vi "04.1 Property Node with Event-driven SM.vi"() -> ()   [LabVIEW 2019]
uses:
  Support Files/02.4 DAQmx Configuration Cluster.ctl
  Support Files/03.2 States.ctl
  Support Files/03.2 State Machine Data.ctl
  <vilib>/DAQmx/write.llb/DAQmx Write (Analog DBL 1Chan 1Samp).vi
  <vilib>/Utility/file.llb/Write Delimited Spreadsheet (string).vi
  <vilib>/Utility/file.llb/Write Delimited Spreadsheet (DBL).vi
  <vilib>/DAQmx/create/channels.llb/DAQmx Create Channel (AO-Voltage-Basic).vi
  <vilib>/DAQmx/miscellaneous.llb/DAQmx Fill In Error Info.vi
panel:
  in  "DAQmx Configuration Cluster":T1={"Desired Sample Rate (Hz)"=-1.0, "sample mode"=10178, "Minimum value"=-1.0, "Maximum value"=-1.0, "Physical Channel"="", "units"=10143, "thermocouple type"=10072, "Samples per Channel"=0} {"thermocouple type" items=["J"=10072, "K"=10073, "N"=10077, "R"=10082, "S"=10085, "T"=10086, "B"=10047, "E"=10055]; "units" items=["Deg C"=10143, "Deg F"=10144, "Kelvins"=10325, "Deg R"=10145, "From Custom Scale"=10065]; "sample mode" items=["Finite Samples"=10178, "Continuous Samples"=10123, "Hardware Timed Single Point"=12522]}
  in  "Threshold (RMS)":dbl
  in  "Generate Stimulus":bool
  in  "Stop":bool
  in  "Clear":bool
  in  "Acquire":bool
  out "Graph":dbl[][](graph)
  out "Thershold Exceeded?":bool
  out "RMS Result per Channel":dbl[](array[numeric])
  # "ANALYSIS"
  # "EVENTS"
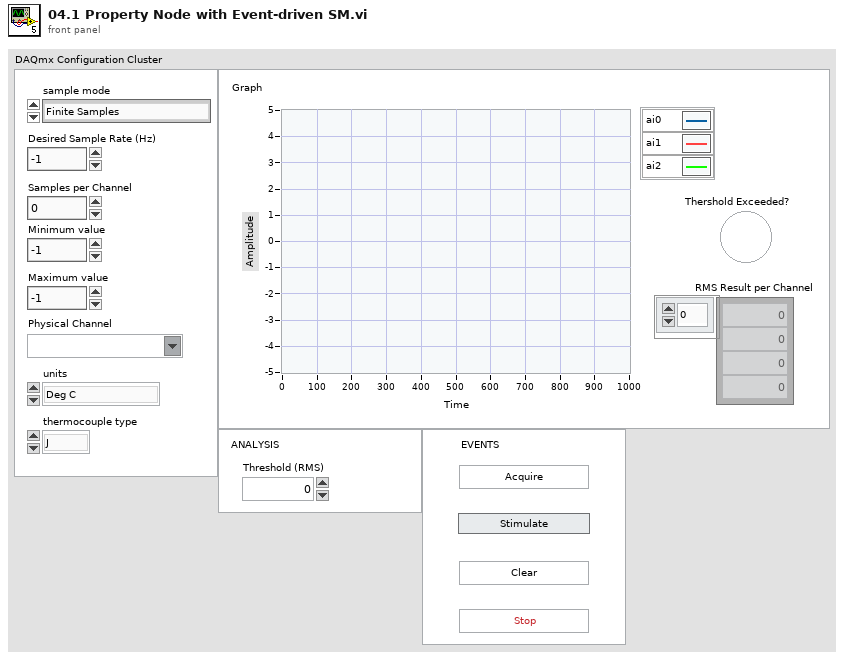
[diagram p1: front panel]
types:
  T1 = typedef "02.4 DAQmx Configuration Cluster.ctl" = cluster{"Desired Sample Rate (Hz)":dbl, "sample mode":i32, "Minimum value":dbl, "Maximum value":dbl, "Physical Channel":tag, "units":i32, "thermocouple type":i32, "Samples per Channel":i32}
  T2 = typedef "03.2 State Machine Data.ctl" = cluster{"Acquisition Data":dbl[][], "Stimulus?":bool}
  T3 = typedef "03.2 States.ctl" = enum16{"Initialize", "Update UI", "Update Stimulus", "Wait for event", "Acquire", "Analyze", "Log", "Clear", "Shutdown"}
  T4 = enum8{"Enabled", "Disabled", "Disabled and Grayed Out"}
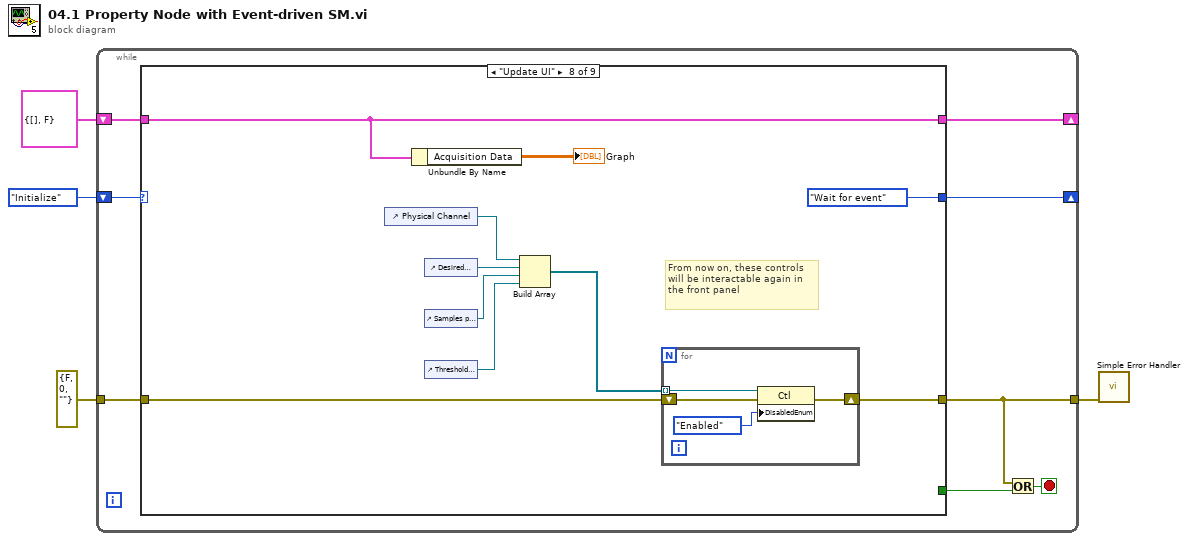
[diagram p0: block diagram]
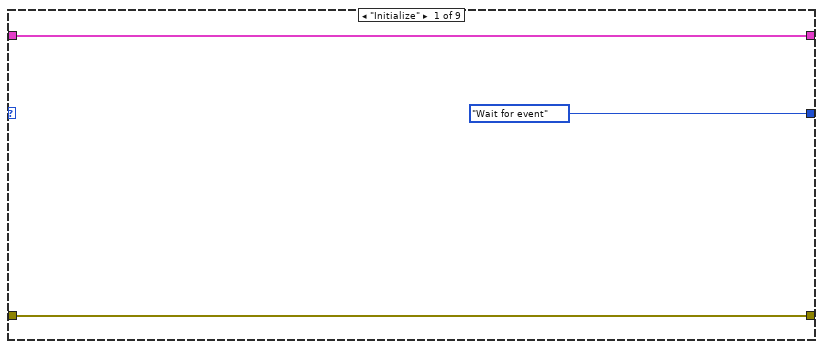
[diagram p2: hidden frame]
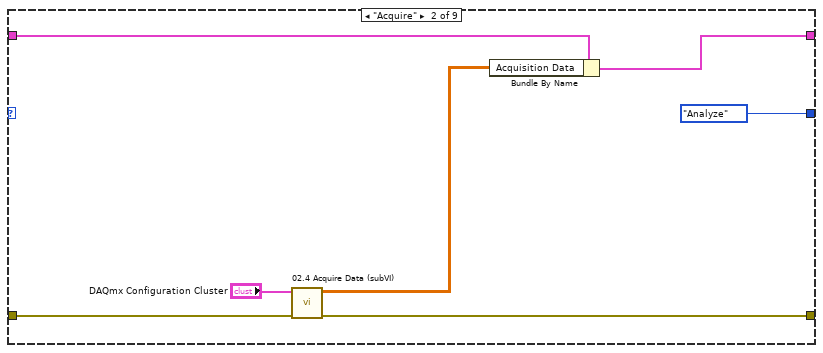
[diagram p3: hidden frame]
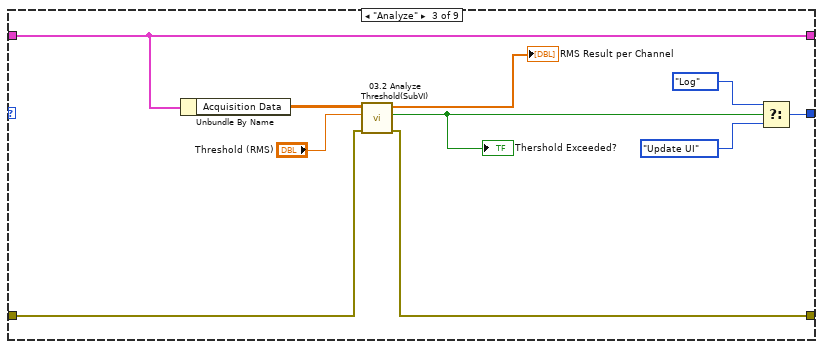
[diagram p4: hidden frame]
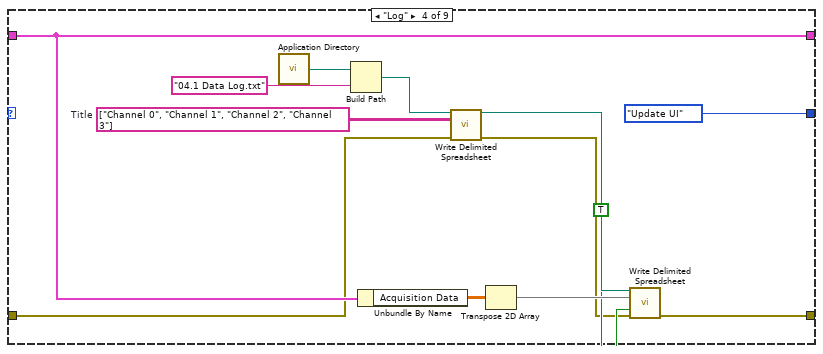
[diagram p5: hidden frame]
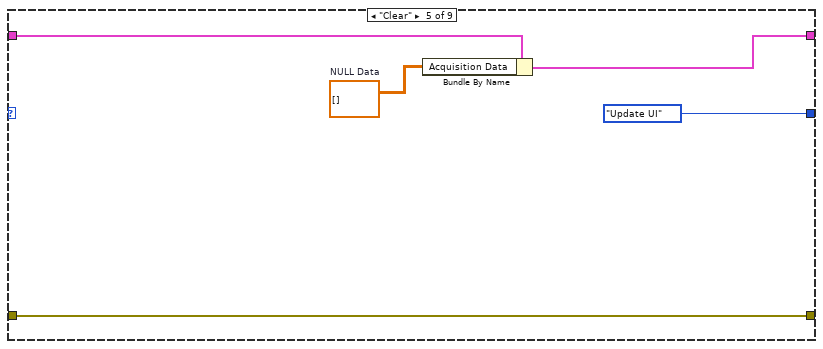
[diagram p6: hidden frame]
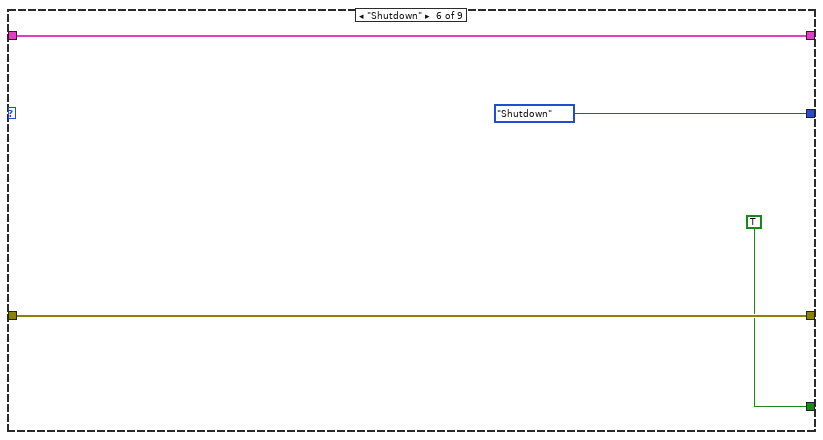
[diagram p7: hidden frame]
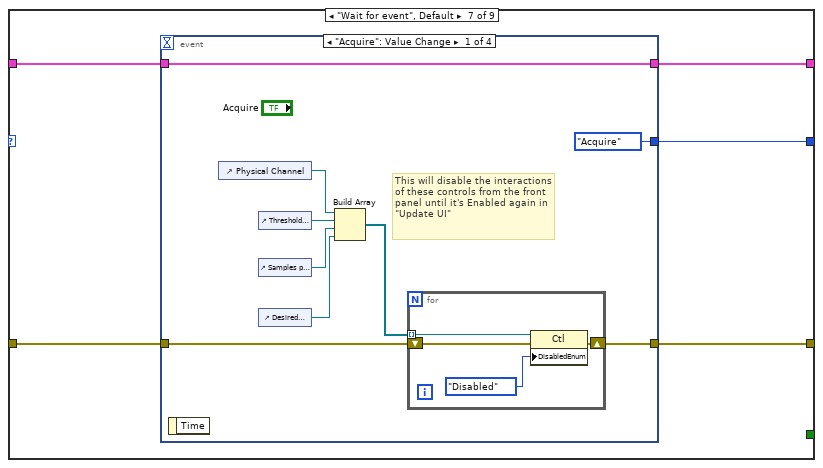
[diagram p8: hidden frame]
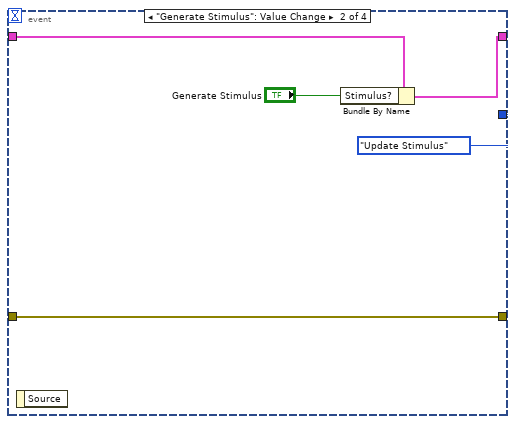
[diagram p9: hidden frame]
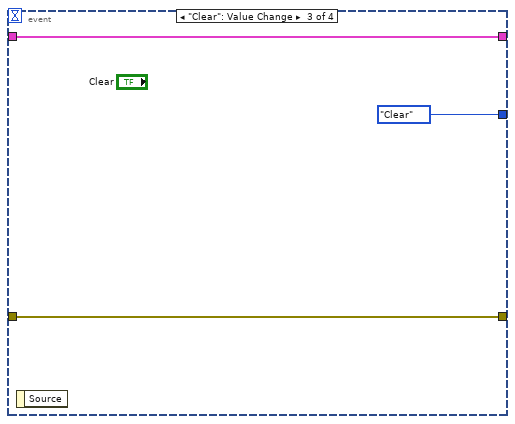
[diagram p10: hidden frame]
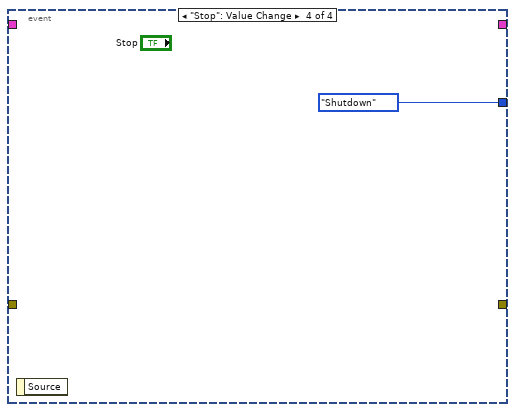
[diagram p11: hidden frame]
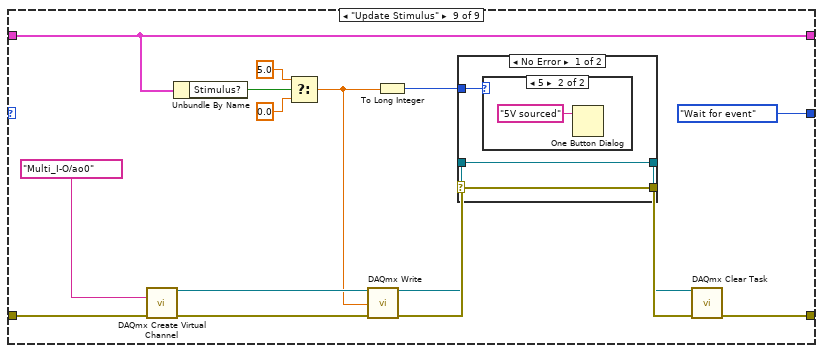
[diagram p12: hidden frame]
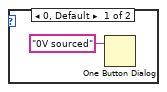
[diagram p13: hidden frame]
diagram:
  n1 = while {
    shift-right: [w11] -> _
    shift-left: 03.2_States."Initialize" ("State") -> [w12]
    tunnel: errorcluster {"status"=FALSE, "code"=0, "source"=""} ("error constant") -> [w10]
    tunnel: [w8] -> w2
    shift-right: [w7] -> _
    shift-left: T2 {"Acquisition Data"=[], "Stimulus?"=FALSE} -> [w6]
    stop <- w9 stop-if-true
    n2 = case shown="\"Update UI\"" w12 {
      tunnel: [03.2_States."Wait for event" ("State") 03.2_States."Analyze" ("State") w31 03.2_States."Update UI" ("State") 03.2_States."Update UI" ("State") 03.2_States."Shutdown" ("State") w59 03.2_States."Wait for event" ("State") 03.2_States."Wait for event" ("State")] -> w11
      tunnel: [w14 w18 w26 w43 w46 w52 w58 w87 w100] -> w8
      tunnel: w10 -> [w14 w19 w27 w33 w46 w52 w57 w86 w111]
      tunnel: [w15 w21 w25 w41 w49 w53 w56 w91 w97] -> w7
      tunnel: w6 -> [w15 w22 w25 w41 w50 w53 w55 w91 w97]
      tunnel: [_ _ _ _ _ TRUE _ _ _] -> w5
      frame "Initialize" {
      }
      frame "Acquire" {
        n3 = call "02.4 Acquire Data (subVI).vi"("Error In"=w19, "DAQmx Configuration Cluster"="DAQmx Configuration Cluster") -> ("error out"=w18:errorcluster, "2D DBL"=w20:dbl[][])  [unwired: 8 in]
        n4 = Bundle By Name(cluster=w22, "Acquisition Data"=w20) -> (w21:T2)
      }
      frame "Analyze" {
        n5 = Unbundle By Name(w25) -> ("Acquisition Data"=w32:dbl[][])
        n6 = call "03.2 Analyze Threshold(SubVI).vi"("Error In"=w27, "Threshold (RMS)"="Threshold (RMS)", "Data"=w32) -> ("Error Out"=w26:errorcluster, "Threshold exceeded?"=w28:bool, "RMS Results per Channel"=→"RMS Result per Channel":dbl[])  [unwired: 6 in]
        "Thershold Exceeded?" <- w28
        n7 = Select(t=03.2_States."Log" ("State"), s=w28, f=03.2_States."Update UI" ("State")) -> (s? t:f=w31:T3)
      }
      frame "Log" {
        w35 = string[][] [["Channel 0", "Channel 1", "Channel 2", "Channel 3"]]  # Title
        n8 = call <vilib>:"Application Directory.vi"() -> ("Application Directory"=w45:path)
        n9 = Build Path(base path=w45, name or relative path="04.1 Data Log.txt") -> (appended path=w36:path)
        n10 = Unbundle By Name(w41) -> ("Acquisition Data"=w40:dbl[][])
        n11 = call-poly <vilib>:"Write Delimited Spreadsheet.vi"("file path (dialog if empty)"=w36, "2D data"=w35, "error in (no error)"=w33) -> ("new file path (Not A Path if cancelled)"=w38:path, "error out"=w34:errorcluster)  [unwired: 11 in]
        n12 = Transpose 2D Array(2D array=w40) -> (transposed array=w39:dbl[][])
        n13 = call-poly <vilib>:"Write Delimited Spreadsheet.vi"("file path (dialog if empty)"=w38, "2D data"=w39, "append to file? (new file:F)"=TRUE, "error in (no error)"=w34) -> ("error out"=w43:errorcluster)  [unwired: 10 in, 1 out]
      }
      frame "Clear" {
        w48 = dbl[][] []  # NULL Data
        n14 = Bundle By Name(cluster=w50, "Acquisition Data"=w48) -> (w49:T2)
      }
      frame "Shutdown" {
      }
      frame "Wait for event", Default {
        n15 = event shown="[0] \"Acquire\": Value Change" {
          selector: _ -> [_ _ _ _]
          dyn-events: _ -> [_ _ _ _]
          timeout: _ -> [_ _ _ _]
          tunnel: [03.2_States."Acquire" ("State") 03.2_States."Update Stimulus" ("State") 03.2_States."Clear" ("State") 03.2_States."Shutdown" ("State")] -> w59
          tunnel: [w60 w73 w78 _] -> w58
          tunnel: w57 -> [w61 w73 w78 _]
          tunnel: [w67 w75 w80 _] -> w56
          tunnel: w55 -> [w67 w77 w80 _]
          event "Acquire": Value Change {
            # "This will disable the interactions of these controls from the front panel until it's Enabled again in \"Update UI\""
            n16 = event-data() -> ()  [unwired: 1 in, 1 out]
            n17 = control-ref of="Physical Channel"() -> (w66:refnum<vi>)
            n18 = control-ref of="Threshold (RMS)"() -> (w65:refnum<vi>)
            n19 = control-ref of="Samples per Channel"() -> (w64:refnum<vi>)
            n20 = control-ref of="Desired Sample Rate (Hz)"() -> (w63:refnum<vi>)
            n21 = Build Array(w66, w65, w64, w63) -> (w62:refnum<vi>[])
            n22 = for {
              tunnel: w62 -> [w72] mode=indexing
              shift-right: [w69] -> w60
              shift-left: w61 -> [w70]
              n23 = property class="Ctl"(reference=w72, error in=w70, "DisabledEnum"=T4."Disabled" ("Disabled")) -> (error out=w69:errorcluster)  [unwired: 1 out]
            }
          }
          event "Generate Stimulus": Value Change {
            n24 = event-data() -> ()  [unwired: 1 in, 1 out]
            n25 = Bundle By Name(cluster=w77, "Stimulus?"="Generate Stimulus") -> (w75:T2)
          }
          event "Clear": Value Change {
            n26 = event-data() -> ()  [unwired: 1 in, 1 out]
          }
          event "Stop": Value Change {
            n27 = event-data() -> ()  [unwired: 1 in, 1 out]
          }
        }
      }
      frame "Update UI" {
        # "From now on, these controls will be interactable again in the front panel"
        n28 = control-ref of="Physical Channel"() -> (w85:refnum<vi>)
        n29 = Unbundle By Name(w91) -> ("Acquisition Data"=→"Graph":dbl[][])
        n30 = control-ref of="Desired Sample Rate (Hz)"() -> (w84:refnum<vi>)
        n31 = control-ref of="Samples per Channel"() -> (w83:refnum<vi>)
        n32 = control-ref of="Threshold (RMS)"() -> (w82:refnum<vi>)
        n33 = Build Array(w85, w84, w83, w82) -> (w88:refnum<vi>[])
        n34 = for {
          tunnel: w88 -> [w95] mode=indexing
          shift-right: [w92] -> w87
          shift-left: w86 -> [w93]
          n35 = property class="Ctl"(reference=w95, error in=w93, "DisabledEnum"=T4."Enabled" ("Disabled")) -> (error out=w92:errorcluster)  [unwired: 1 out]
        }
      }
      frame "Update Stimulus" {
        n36 = call-poly <vilib>:"DAQmx Create Virtual Channel.vi"("physical channels"=tag "Multi_I-O/ao0", "error in"=w111) -> ("task out"=w109:refnum<k21>, "error out"=w110:errorcluster)  [unwired: 12 in]
        n37 = Unbundle By Name(w97) -> ("Stimulus?"=w108:bool)
        n38 = Select(t=5.0, s=w108, f=0.0) -> (s? t:f=w105:dbl)
        n39 = call-poly <vilib>:"DAQmx Write.vi"("task/channels in"=w109, "data"=w105, "error in"=w110) -> ("task out"=w103:refnum<k21>, "error out"=w104:errorcluster)  [unwired: 10 in, 1 out]
        n40 = To Long Integer(number=w105) -> (32bit integer=w98:i32)
        n41 = case shown="No Error" w104 {
          selector: w104 -> [w114 w117]
          tunnel: w103 -> [w113 w118]
          tunnel: [w114 w117] -> w102
          tunnel: [w113 w118] -> w101
          tunnel: w98 -> [w112 _]
          frame No Error {
            n42 = case shown="5" w112 {
              frame 0, Default {
                n43 = One Button Dialog(message="0V sourced") -> ()  [unwired: 1 in, 1 out]
              }
              frame 5 {
                n44 = One Button Dialog(message="5V sourced") -> ()  [unwired: 1 in, 1 out]
              }
            }
          }
          frame Error {
          }
        }
        n45 = call <vilib>:"DAQmx Clear Task.vi"("task in"=w101, "error in"=w102) -> ("error out"=w100:errorcluster)  [unwired: 13 in]
      }
    }
    n46 = Or(x=w8, y=w5) -> (x .or. y?=w9:bool)
  }
  n47 = call <vilib>:"Simple Error Handler.vi"("error in (no error)"=w2) -> ()  [unwired: 4 in, 5 out]
